vi "PackType.vi"() -> ()   [LabVIEW 2020]
panel:
  out "VG_PackType":string
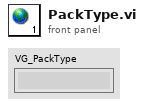
[diagram p1: front panel]
diagram:
